vi "Manual Set LVDT's.vi"(9 "LVDT Numbers":i32[](array[numeric]), 10 "Data":dbl[](array[numeric]) min=-50.0 max=50.0 format="%.1f", 11 "LVDT's 1":refnum<visa-resource-name>="COM1") -> (0 "Error":errorcluster, 3 "appended array 2":string[](array[string]))   [LabVIEW 2018]
uses:
  <vilib>/Instr/_visa.llb/VISA Configure Serial Port (Instr).vi
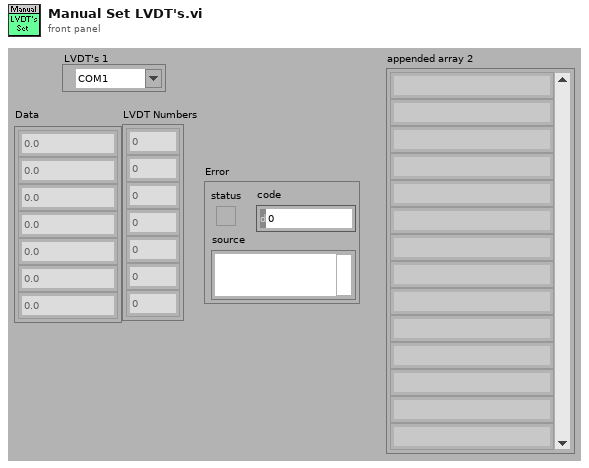
[diagram p1: front panel]
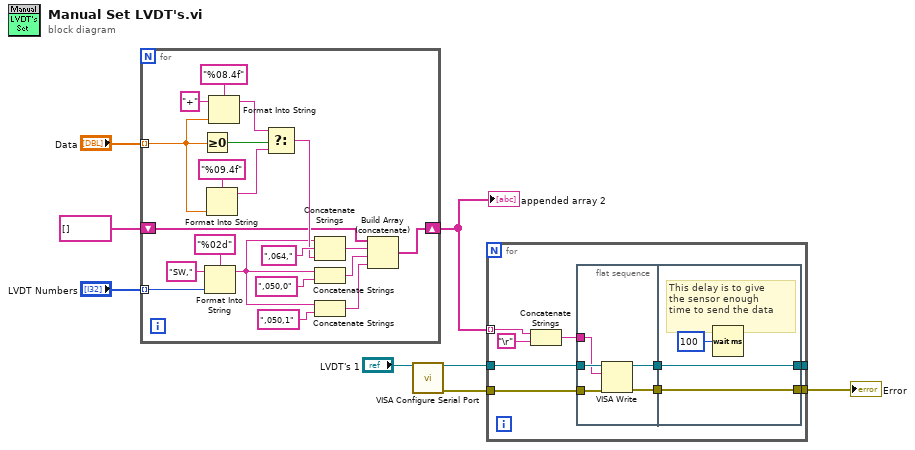
[diagram p0: block diagram]
diagram:
  n1 = for {
    tunnel: "Data" -> [w11] mode=indexing
    shift-right: [w12] -> w8
    shift-left: string[] [] -> [w10]
    tunnel: "LVDT Numbers" -> [w9] mode=indexing
    n2 = Greater Or Equal To 0?(x=w11) -> (x >= 0?=w26:bool)
    n3 = Format Into String(format string="%02d", initial string="SW,", w9) -> (resulting string=w17:string)  [unwired: 1 in, 1 out]
    n4 = Format Into String(format string="%09.4f", w11) -> (resulting string=w23:string)  [unwired: 2 in, 1 out]
    n5 = Format Into String(format string="%08.4f", initial string="+", w11) -> (resulting string=w25:string)  [unwired: 1 in, 1 out]
    n6 = Select(t=w25, s=w26, f=w23) -> (s? t:f=w20:string)
    n7 = Concatenate Strings(w17, ",064," ("write buffer"), w20) -> (w16:string)
    n8 = Concatenate Strings(w17, ",050,0" ("write buffer")) -> (w15:string)
    n9 = Concatenate Strings(w17, ",050,1" ("write buffer")) -> (w14:string)
    n10 = Build Array (concatenate)(w10, w16, w15, w14) -> (w12:string[])
  }
  "appended array 2" <- w8
  n11 = call-poly "VISA Configure Serial Port"("VISA resource name"="LVDT's 1") -> ("VISA resource name out"=w3:refnum<visa-resource-name>, "error out"=w1:errorcluster)  [unwired: 13 in]
  n12 = for {
    tunnel: w3 -> [w34]
    tunnel: [w33] -> w2
    tunnel: [w32] -> _
    tunnel: w8 -> [w30] mode=indexing
    tunnel: w1 -> [w29]
    n13 = Concatenate Strings(w30, "\r") -> (w35:string)
    n14 = flat-sequence {
      tunnel: w34 -> [w42]
      tunnel: w35 -> [w38]
      tunnel: [w41] -> w37
      tunnel: [w40] -> w36
      tunnel: w29 -> [w39]
      tunnel: [w44] -> w32
      tunnel: w37 -> [w44]
      tunnel: [w43] -> w33
      tunnel: w36 -> [w43]
      frame #0 {
        n15 = VISA Write(VISA resource name=w42, write buffer=w38, error in (no error)=w39) -> (VISA resource name out=w41:refnum<visa-resource-name>, error out=w40:errorcluster)  [unwired: 1 out]
      }
      frame #1 {
        # "This delay is to give\nthe sensor enough\ntime to send the data"
        n16 = Wait (ms)(milliseconds to wait=u32 100) -> ()  [unwired: 1 out]
      }
    }
  }
  "Error" <- w2
